vi "Error Beep.vi"   [LabVIEW 2014]
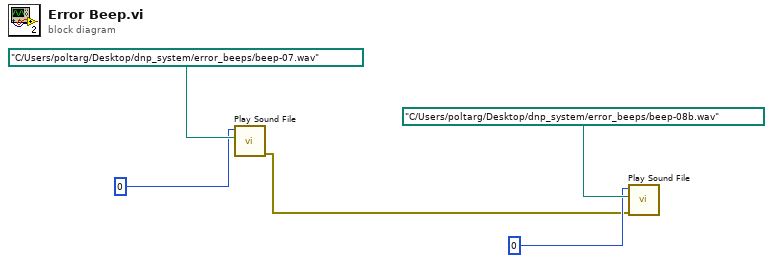
[diagram p0: block diagram]
diagram:
  n1 = call <vilib>:"Play Sound File.vi"("path"=path "C:/Users/poltarg/Desktop/dnp_system/error_beeps/beep-07.wav", "device ID"=0) -> ("error out"=w1:errorcluster)  [unwired: 8 in, 1 out]
  n2 = call <vilib>:"Play Sound File.vi"("error in (no error)"=w1, "path"=path "C:/Users/poltarg/Desktop/dnp_system/error_beeps/beep-08b.wav", "device ID"=0) -> ()  [unwired: 7 in, 2 out]
